vi "Calibration Models Comparison Processing.vi"(8 "error in (no error)":errorcluster, 10 "Temp Image":T1, 11 "Test Image":T1) -> (0 "error out":errorcluster, 1 "Elapsed Time (ms)":dbl, 2 "Results":sgl[](array[numeric]), 3 "Test Image Out":T1)   [LabVIEW 2014]
doc: "This processing subVI locates the object in the scene, and measure the part height in 50 different locations."
uses:
  <vilib>/vision/Image Controls.llb/IMAQ Image.ctl
  <vilib>/vision/Measure.llb/Edge Options.ctl
  <vilib>/vision/Measure.llb/Edge Polarity.ctl
  <vilib>/vision/NI_Vision_Development_Module.lvlib
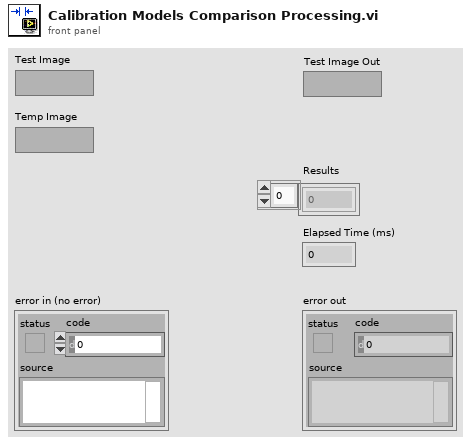
[diagram p1: front panel]
types:
  T1 = typedef "IMAQ Image.ctl" = refnum<image>
  T2 = cluster{"Area":dbl, "Number of Holes":dbl, "Bounding Rect":cluster{"Left":dbl, "Top":dbl, "Right":dbl, "Bottom":dbl}, "Center of Mass":cluster{"X":dbl, "Y":dbl}, "Orientation":dbl, "Dimensions":cluster{"Width":dbl, "Height":dbl}}[]
  T3 = cluster{"Area":dbl, "Number of Holes":dbl, "Bounding Rect":cluster{"Left":dbl, "Top":dbl, "Right":dbl, "Bottom":dbl}, "Center of Mass":cluster{"X":dbl, "Y":dbl}, "Orientation":dbl, "Dimensions":cluster{"Width":dbl, "Height":dbl}}
  T4 = cluster{"Left":dbl, "Top":dbl, "Right":dbl, "Bottom":dbl}
  T5 = enum16{"Get First Edge", "Get First + Last Edge", "Get All Edges", "Get Best Edge"}
  T6 = typedef "Edge Options.ctl" = cluster{"Edge Polarity":T7, "Kernel Size":u32, "Width":u32, "Minimum Edge Strength":sgl, "Interpolation Type":enum32{"Zero Order", "Bilinear", "Quadratic", "Cubic", "Bilinear Fixed"}, "Data Processing Method":enum32{"Average", "Median"}}
  T7 = typedef "Edge Polarity.ctl" = u32
  T8 = typedef "ROI Descriptor" = cluster{"Global Rectangle":i32[], "Contours":cluster{"ID":enum32{"External", "Internal"}, "Type":u32, "Coordinates":i32[]}[]}
  T9 = typedef "Edge New.ctl" = cluster{"Location (Pixel)":cluster{"X":sgl, "Y":sgl}, "Location (Real-World)":cluster{"X":sgl, "Y":sgl}, "Distance (Pixel)":dbl, "Distance (Real-World)":dbl, "Strength":dbl, "Noise":dbl, "Rising?":bool}
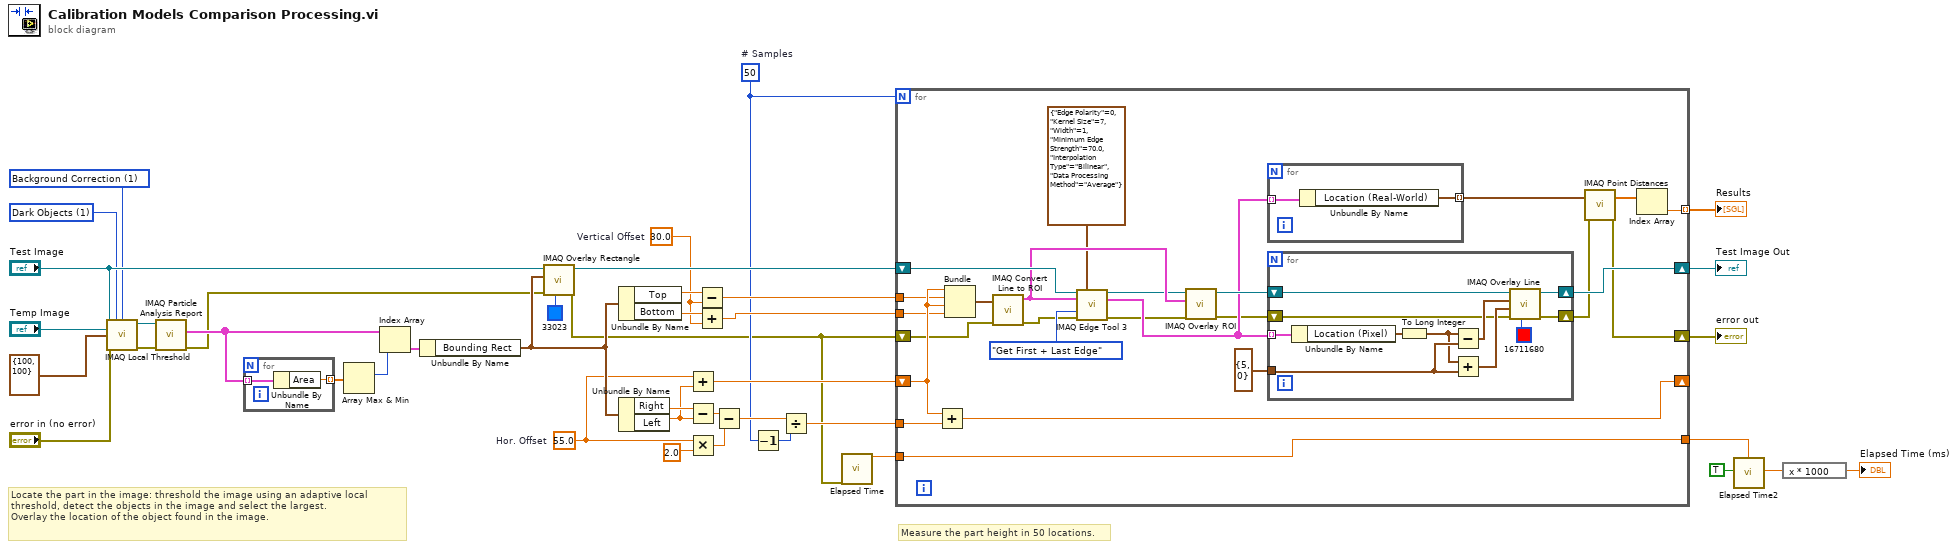
[diagram p0: block diagram]
diagram:
  w13 = 50  # # Samples
  w17 = 30.0  # Vertical Offset
  w11 = 55.0  # Hor. Offset
  w28 = u32 1 items=["Niblack", "Background Correction"] ("Method (Niblack)")
  w29 = u32 1 items=["Bright Objects", "Dark Objects"] ("Look For (Bright Objects)")
  # "Measure the part height in 50 locations."
  # "Locate the part in the image: threshold the image using an adaptive local threshold, detect the objects in the image and select the largest.\nOverlay the location of the object found in the image."
  n1 = call "IMAQ Local Threshold"("Image Src"="Test Image", "Look For (Bright Objects)"=w29, "Method (Niblack)"=w28, "Image Dst"="Temp Image", "Window Size (32x32)"=cluster{"SizeX":i32, "SizeY":i32} {"SizeX"=100, "SizeY"=100}, "error in (no error)"="error in (no error)") -> ("Image Dst Out"=w26:T1, "error out"=w9:errorcluster)  [unwired: 2 in, 6 out]
  n2 = call "IMAQ Particle Analysis Report"("error in (no error)"=w9, "Image"=w26) -> ("error out"=w8:errorcluster, "Particle Reports (Pixels)"=w32:T2)  [unwired: 1 in, 7 out]
  n3 = for {
    tunnel: w32 -> [w43] mode=indexing
    tunnel: [w42] -> w31 mode=indexing
    n4 = Unbundle By Name(w43) -> ("Area"=w42:dbl)
  }
  n5 = Array Max & Min(array=w31) -> (max index (indices)=w30:i32)  [unwired: 3 out]
  n6 = Index Array(array=w32, index=w30) -> (element=w34:T3)
  n7 = Unbundle By Name(w34) -> ("Bounding Rect"=w36:T4)
  n8 = call "IMAQ Overlay Rectangle"("Color"=u32 33023, "error in (no error)"=w8, "Rectangle"=w36, "Image"="Test Image") -> ("error out"=w1:errorcluster, "Image Out"=w35:T1)  [unwired: 2 in, 4 out]
  n9 = Unbundle By Name(w36) -> ("Top"=w19:dbl, "Bottom"=w18:dbl)
  n10 = Unbundle By Name(w36) -> ("Right"=w25:dbl, "Left"=w21:dbl)
  n11 = Add(x=w11, y=w21) -> (x+y=w20:dbl)
  n12 = Subtract(x=w25, y=w21) -> (x-y=w24:dbl)
  n13 = Multiply(x=w11, y=2.0) -> (x*y=w22:dbl)
  n14 = Subtract(x=w19, y=w17) -> (x-y=w16:dbl)
  n15 = Add(x=w18, y=w17) -> (x+y=w15:dbl)
  n16 = Subtract(x=w24, y=w22) -> (x-y=w14:dbl)
  n17 = Decrement(x=w13) -> (x-1=w12:i32)
  n18 = Divide(x=w14, y=w12) -> (x/y=w7:dbl)
  n19 = call "Elapsed Time"("error in (no error)"=w1) -> ("Present (s)"=w2:dbl)  [unwired: 11 in, 7 out]
  n20 = for {
    N: w13 -> [_]
    shift-right: [w51] -> _
    shift-left: w20 -> [w68]
    tunnel: w16 -> [w67]
    tunnel: w15 -> [w66]
    tunnel: w7 -> [w65]
    shift-right: [w64] -> w38
    shift-left: w35 -> [w63]
    tunnel: [w62] -> w39 mode=indexing
    shift-right: [w46] -> w37
    shift-left: w1 -> [w45]
    tunnel: w2 -> [w44]
    tunnel: [w44] -> w4
    n21 = Add(x=w68, y=w65) -> (x+y=w51:dbl)
    n22 = Bundle(w68, w67, w68, w66) -> (w60:cluster{dbl, dbl, dbl, dbl})  [unwired: 1 out]
    n23 = call "IMAQ Convert Line to ROI"("error in (no error)"=w45, "Line"=w60) -> ("error out"=w50:errorcluster, "ROI Descriptor"=w61:T8)  [unwired: 7 out]
    n24 = call "IMAQ Edge Tool 3"("Image"=w63, "Edge Options"=T6 {"Edge Polarity"=0, "Kernel Size"=7, "Width"=1, "Minimum Edge Strength"=70.0, "Interpolation Type"=enum."Bilinear", "Data Processing Method"=enum."Average"}, "ROI Descriptor"=w61, "Process"=T5."Get First + Last Edge", "error in (no error)"=w50) -> ("Image (duplicate)"=w53:T1, "Edge Information"=w52:T9[], "error out"=w49:errorcluster)  [unwired: 2 in, 6 out]
    n25 = call "IMAQ Overlay ROI"("error in (no error)"=w49, "ROI Descriptor"=w61, "Image"=w53) -> ("error out"=w48:errorcluster, "Image Out"=w55:T1)  [unwired: 3 in, 4 out]
    n26 = for {
      tunnel: w52 -> [w81] mode=indexing
      tunnel: [w80] -> w57 mode=indexing
      n27 = Unbundle By Name(w81) -> ("Location (Real-World)"=w80:cluster{"X":sgl, "Y":sgl})
    }
    n28 = for {
      tunnel: w52 -> [w79] mode=indexing
      shift-right: [w77] -> w64
      shift-left: w55 -> [w78]
      tunnel: cluster{"X":i32, "Y":i32} {"X"=5, "Y"=0} ("y") -> [w73]
      shift-right: [w69] -> w47
      shift-left: w48 -> [w70]
      n29 = Unbundle By Name(w79) -> ("Location (Pixel)"=w75:cluster{"X":sgl, "Y":sgl})
      n30 = To Long Integer(number=w75) -> (32bit integer=w71:cluster{"X":i32, "Y":i32})
      n31 = Subtract(x=w71, y=w73) -> (x-y=w76:cluster{"X":i32, "Y":i32})
      n32 = Add(x=w71, y=w73) -> (x+y=w74:cluster{"X":i32, "Y":i32})
      n33 = call "IMAQ Overlay Line"("Color"=u32 16711680, "error in (no error)"=w70, "End Point"=w74, "Start Point"=w76, "Image"=w78) -> ("error out"=w69:errorcluster, "Image Out"=w77:T1)  [unwired: 1 in, 4 out]
    }
    n34 = call "IMAQ Point Distances"("Points"=w57, "error in (no error)"=w47) -> ("Distances"=w56:sgl[], "error out"=w46:errorcluster)  [unwired: 3 out]
    n35 = Index Array(array=w56) -> (element=w62:sgl)  [unwired: 1 in]
  }
  "Results" <- w39
  "Test Image Out" <- w38
  "error out" <- w37
  n36 = call "Elapsed Time2"("Reset"=TRUE, "Set Start Time (s)"=w4) -> ("Elapsed Time (s)"=w5:dbl)  [unwired: 10 in, 7 out]
  n37 = expression code="x * 1000"(w5) -> (→"Elapsed Time (ms)":dbl)
